vi "rawpathToInterp.vi"(8 "error in (no error)":errorcluster, 10 "create interp img folder":bool=TRUE, 11 "Path":path) -> (0 "error out":errorcluster, 1 "Angle lineout path":path, 2 "Spectrum lineout path":path, 3 "Interpolated image path":path)   [LabVIEW 2013]
panel:
  out "Interp folder":path
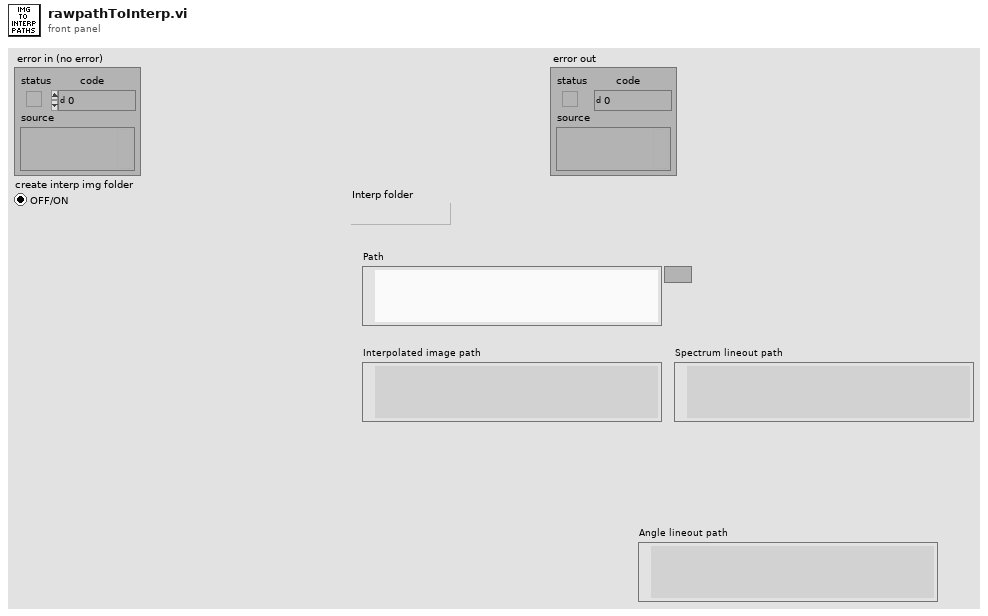
[diagram p1: front panel]
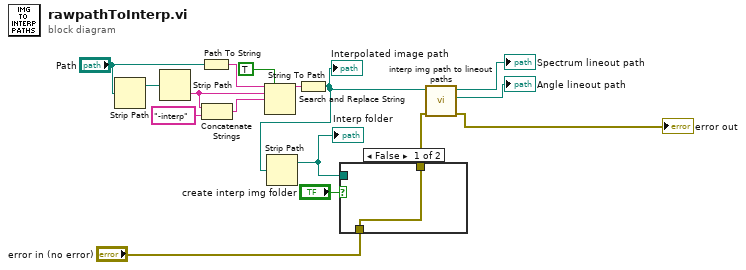
[diagram p0: block diagram]
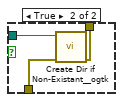
[diagram p2: hidden frame]
diagram:
  n1 = Strip Path(path="Path") -> (stripped path=w15:path)  [unwired: 1 out]
  n2 = Strip Path(path=w15) -> (name=w12:string)  [unwired: 1 out]
  n3 = Path To String(path="Path") -> (string=w13:string)
  n4 = Concatenate Strings(w12, "-interp") -> (w8:string)
  n5 = Search and Replace String(replace all?=TRUE ("replace all? (F)"), input string=w13, search string=w12, replace string=w8) -> (result string=w10:string)  [unwired: 4 in, 3 out]
  n6 = String To Path(string=w10) -> (path=w2:path)
  "Interpolated image path" <- w2
  n7 = Strip Path(path=w2) -> (stripped path=w5:path)  [unwired: 1 out]
  "Interp folder" <- w5
  n8 = case shown="False" "create interp img folder" {
    tunnel: w5 -> [_ w20]
    tunnel: "error in (no error)" -> [w17 w19]
    tunnel: [w17 w18] -> w3
    frame False {
    }
    frame True {
      n9 = call "Create Dir if Non-Existant__ogtk.vi"("error in (no error)"=w19, "Directory Path"=w20) -> ("error out"=w18:errorcluster)  [unwired: 7 in, 2 out]
    }
  }
  n10 = call "interp img path to lineout paths.vi"("error in (no error)"=w3, "Interp image path"=w2) -> ("error out"=→"error out":errorcluster, "angle lineout path"=→"Angle lineout path":path, "Spectrum lineout path"=→"Spectrum lineout path":path)  [unwired: 7 in]
